vi "multiply_additional_soft_limits.vi"(0 "MotorSystem 输入":refnum<class "MotorSystem.lvclass">, 5 "additional soft limit in":T1(array[cluster]), 7 "dim index":u32, 9 "ratio":dbl, 11 "error in (no error)":errorcluster caption="错误输入（无错误）") -> (4 "MotorSystem 输出":refnum<class "MotorSystem.lvclass">, 6 "additional soft limit out":T1(array[cluster]), 15 "error out":errorcluster caption="错误输出")   [LabVIEW 2016, in "MotionControl_UFO_3DOF.lvlib" / "MotorSystem.lvclass"]
uses:
  <userlib>/MotionControl_UFO_3DOF/MotorSystem/MotorSystem.lvclass
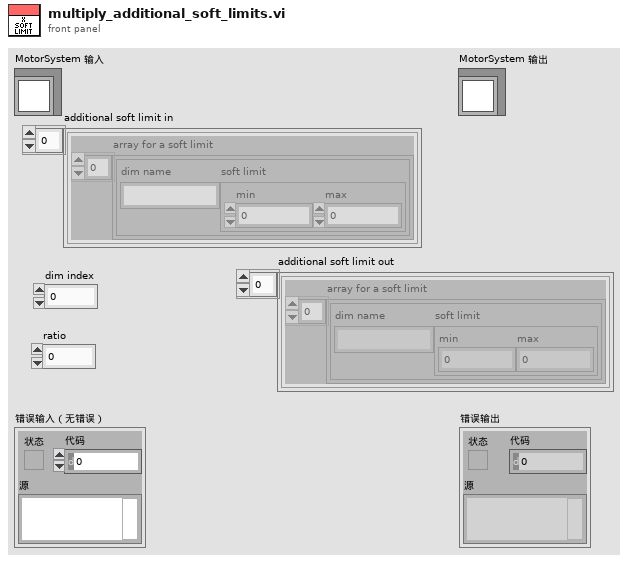
[diagram p1: front panel]
types:
  T1 = cluster{"array for a soft limit":cluster{"dim name":string, "soft limit":cluster{"min":dbl, "max":dbl}}[]}[]
  T2 = cluster{"dim name":string, "soft limit":cluster{"min":dbl, "max":dbl}}[]
  T3 = cluster{"dim name":string, "soft limit":cluster{"min":dbl, "max":dbl}}
  T4 = cluster{"array for a soft limit":cluster{"dim name":string, "soft limit":cluster{"min":dbl, "max":dbl}}[]}
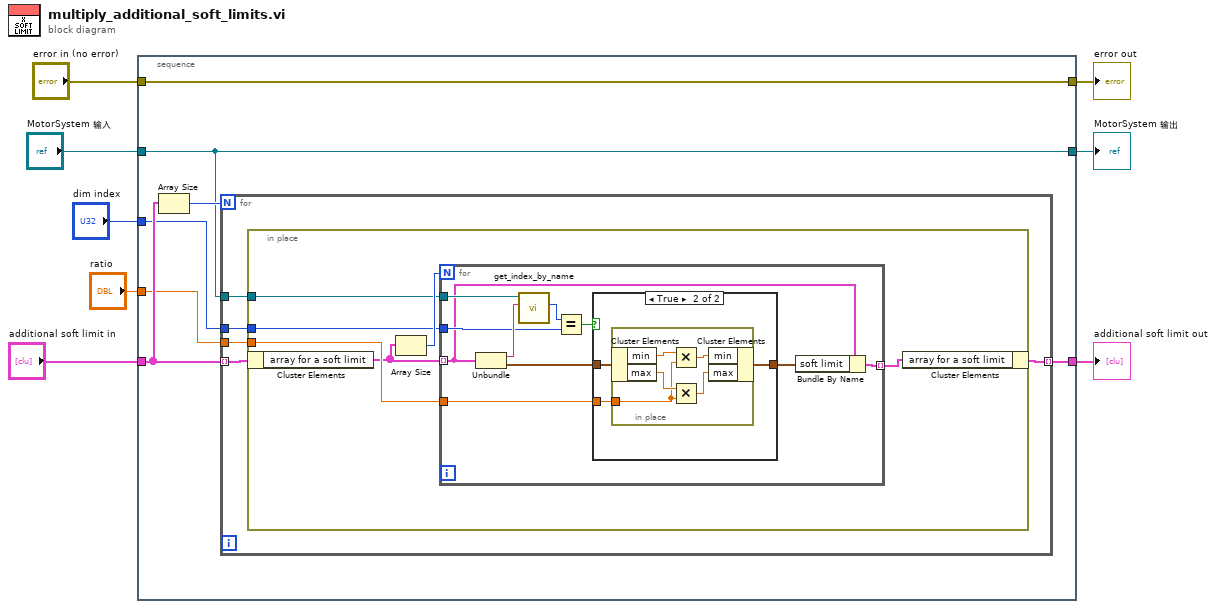
[diagram p0: block diagram]
diagram:
  n1 = stacked-sequence {
    tunnel: [w9] -> w8
    tunnel: [w11] -> w6
    tunnel: "MotorSystem 输入" -> [w11]
    tunnel: "additional soft limit in" -> [w14]
    tunnel: "dim index" -> [w13]
    tunnel: "ratio" -> [w12]
    tunnel: [w10] -> w2
    tunnel: "error in (no error)" -> [w9]
    frame #0 {
      n2 = Array Size(array=w14) -> (size(s)=w15:i32)
      n3 = for {
        N: w15 -> [_]
        tunnel: w14 -> [w17] mode=indexing
        tunnel: w11 -> [w20]
        tunnel: w13 -> [w19]
        tunnel: w12 -> [w18]
        tunnel: [w16] -> w10 mode=indexing
        n4 = in-place {
          in-place-border: w20 -> [w25]
          in-place-border: w19 -> [w24]
          in-place-border: w18 -> [w23]
          n5 = in-place-cluster #1(w17) -> ("array for a soft limit"=w22:T2)
          n6 = Array Size(array=w22) -> (size(s)=w26:i32)
          n7 = for {
            N: w26 -> [_]
            tunnel: w22 -> [w29] mode=indexing
            tunnel: w25 -> [w36]
            tunnel: w24 -> [w33]
            tunnel: w23 -> [w30]
            tunnel: [w27] -> w21 mode=indexing
            n8 = Unbundle(w29) -> ("dim name"=w35:string, "soft limit"=w31:cluster{"min":dbl, "max":dbl})
            n9 = call <userlib>:"get_index_by_name.vi"("name"=w35, "MotorSystem 输入"=w36) -> ("index (0-based)"=w34:u32)  [unwired: 7 in, 2 out]
            n10 = Equal?(x=w34, y=w33) -> (x = y?=w32:bool)
            n11 = case shown="True" w32 {
              tunnel: w31 -> [w37 w40]
              tunnel: w30 -> [_ w39]
              tunnel: [w37 w38] -> w28
              frame False {
              }
              frame True {
                n12 = in-place {
                  in-place-border: w39 -> [w43]
                  n13 = in-place-cluster #2(w40) -> ("min"=w45:dbl, "max"=w44:dbl)
                  n14 = Multiply(x=w45, y=w43) -> (x*y=w42:dbl)
                  n15 = Multiply(x=w44, y=w43) -> (x*y=w41:dbl)
                  n16 = in-place-cluster #2("min"=w42, "max"=w41) -> (w38:cluster{"min":dbl, "max":dbl})
                }
              }
            }
            n17 = Bundle By Name(cluster=w29, "soft limit"=w28) -> (w27:T3)
          }
          n18 = in-place-cluster #1("array for a soft limit"=w21) -> (w16:T4)
        }
      }
    }
  }
  "error out" <- w8
  "MotorSystem 输出" <- w6
  "additional soft limit out" <- w2
